vi "PAQmem_WriteAll.vi"(8 "error in (no error)":errorcluster, 10 "BinHistData":T1, 11 "PAQ-memory in":refnum<class "PAQ-memory.lvclass">) -> (0 "error out":errorcluster, 3 "PAQ-memory out":refnum<class "PAQ-memory.lvclass">)   [LabVIEW 2020, in "PAQ-memory.lvclass"]
doc: "PAQ memory action: write one whole layer content (of multiple TAGs)\n\nThis VI writes fetched data from the database to the computer memory DVR element"
uses:
  PAQ-memory.lvclass
  DBAL/controls/BIN/BINdata.ctl
  PAQ-memory.lvclass/PAQ-memory.ctl
  DBAL/DBAL-BIN.lvclass
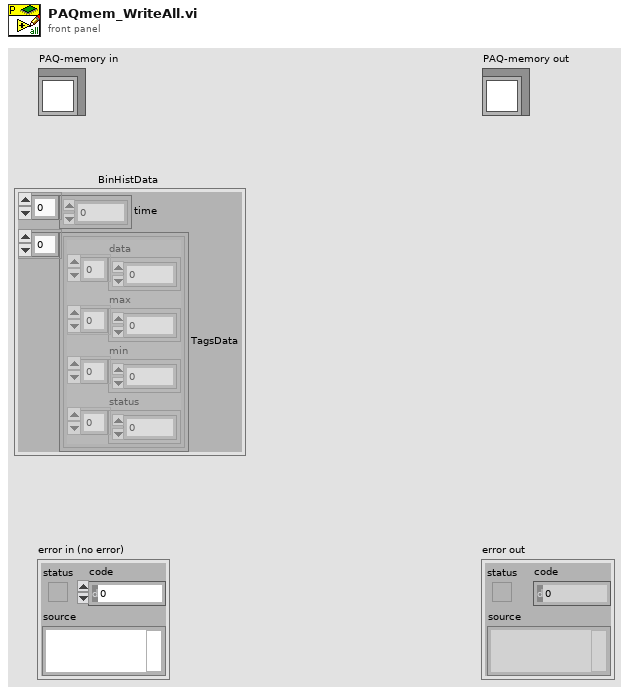
[diagram p1: front panel]
types:
  T1 = typedef "DBAL-BIN.lvclass/BINdata.ctl" = cluster{"time":dbl[], "TagsData":cluster{"data":dbl[], "max":dbl[], "min":dbl[], "status":u32[]}[]}
  T2 = cluster{"data":dbl[], "max":dbl[], "min":dbl[], "status":u32[]}[]
  T3 = cluster{"source":refnum<data-value>, "status":refnum<data-value>, "data":refnum<data-value>, "max":refnum<data-value>, "min":refnum<data-value>}[]
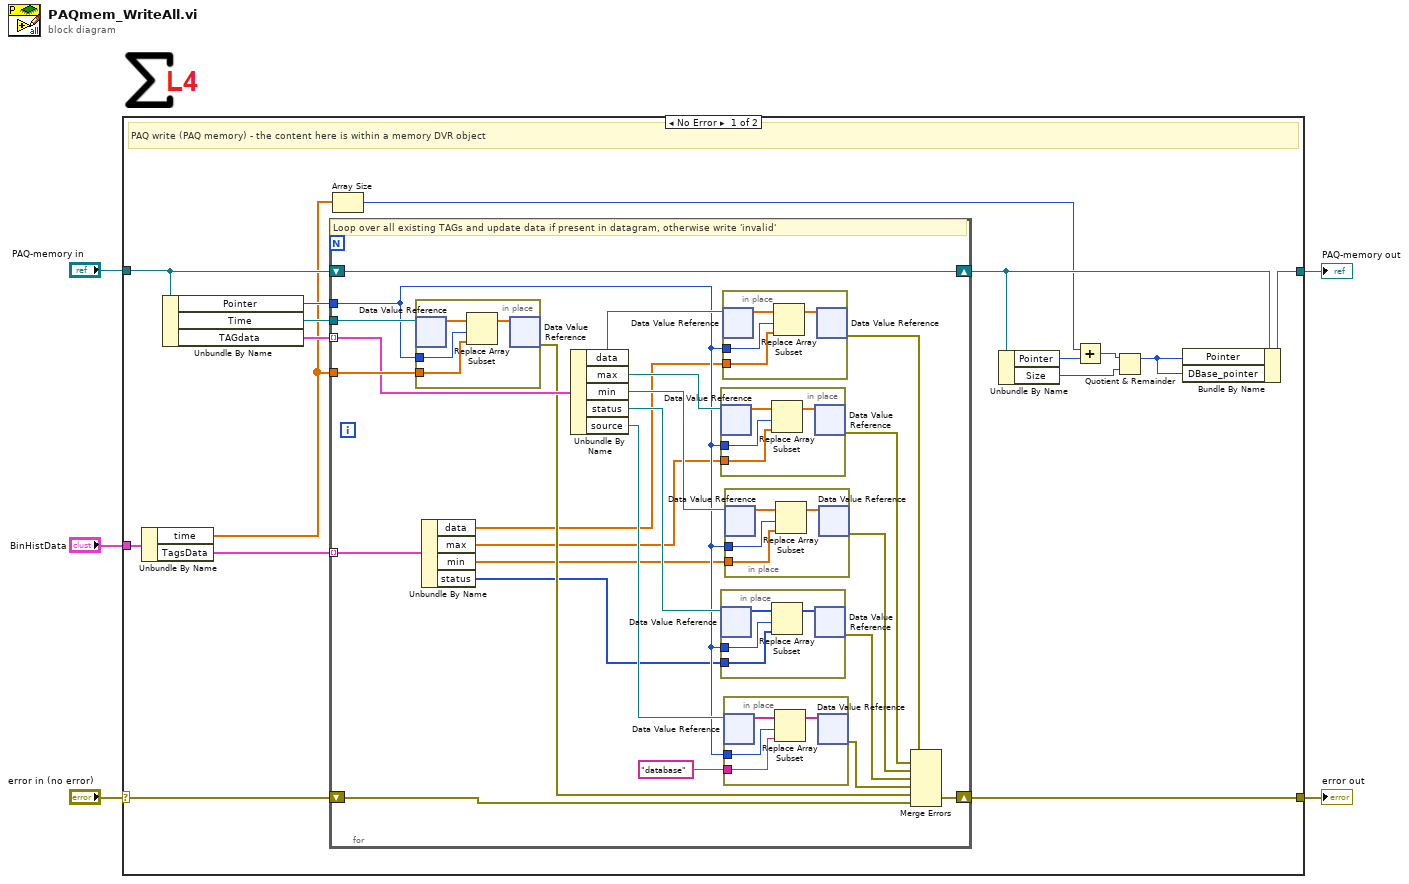
[diagram p0: block diagram]
diagram:
  n1 = case shown="No Error" "error in (no error)" {
    selector: "error in (no error)" -> [w21 w71]
    tunnel: [w20 w71] -> w4
    tunnel: [w13 w70] -> w2
    tunnel: "PAQ-memory in" -> [w19 w70]
    tunnel: "BinHistData" -> [w12 _]
    frame No Error {
      # "PAQ write (PAQ memory) - the content here is within a memory DVR object"
      n2 = Unbundle By Name(w12) -> ("time"=w10:dbl[], "TagsData"=w11:T2)
      n3 = Unbundle By Name(w19) -> ("Pointer"=w18:i32, "Time"=w17:refnum<data-value>, "TAGdata"=w16:T3)
      n4 = for {
        tunnel: w10 -> [w43]
        shift-right: [w33] -> w20
        shift-left: w21 -> [w35]
        shift-right: [w45] -> w14
        shift-left: w19 -> [w45]
        tunnel: w18 -> [w36]
        tunnel: w17 -> [w44]
        tunnel: w16 -> [w42] mode=indexing
        tunnel: w11 -> [w26] mode=indexing
        # "Loop over all existing TAGs and update data if present in datagram, otherwise write 'invalid'"
        n5 = in-place {
          in-place-border: w36 -> [w67]
          in-place-border: w43 -> [w66]
          n6 = in-place-dvr #1(w44) -> (w69:dbl[])  [unwired: 1 out]
          n7 = Replace Array Subset(array=w69, new element=w66, index=w67) -> (w68:dbl[])
          n8 = in-place-dvr #1(w68) -> (w28:errorcluster)  [unwired: 1 out]
        }
        n9 = Unbundle By Name(w26) -> ("data"=w25:dbl[], "max"=w24:dbl[], "min"=w23:dbl[], "status"=w22:u32[])
        n10 = Unbundle By Name(w42) -> ("data"=w41:refnum<data-value>, "max"=w40:refnum<data-value>, "min"=w39:refnum<data-value>, "status"=w38:refnum<data-value>, "source"=w37:refnum<data-value>)
        n11 = in-place {
          in-place-border: w36 -> [w59]
          in-place-border: w24 -> [w58]
          n12 = in-place-dvr #2(w40) -> (w61:dbl[])  [unwired: 1 out]
          n13 = Replace Array Subset(array=w61, new element=w58, index=w59) -> (w60:dbl[])
          n14 = in-place-dvr #2(w60) -> (w32:errorcluster)  [unwired: 1 out]
        }
        n15 = in-place {
          in-place-border: w36 -> [w51]
          in-place-border: w22 -> [w50]
          n16 = in-place-dvr #3(w38) -> (w53:u32[])  [unwired: 1 out]
          n17 = Replace Array Subset(array=w53, new element=w50, index=w51) -> (w52:u32[])
          n18 = in-place-dvr #3(w52) -> (w30:errorcluster)  [unwired: 1 out]
        }
        n19 = in-place {
          in-place-border: w36 -> [w63]
          in-place-border: w25 -> [w62]
          n20 = in-place-dvr #4(w41) -> (w65:dbl[])  [unwired: 1 out]
          n21 = Replace Array Subset(array=w65, new element=w62, index=w63) -> (w64:dbl[])
          n22 = in-place-dvr #4(w64) -> (w34:errorcluster)  [unwired: 1 out]
        }
        n23 = in-place {
          in-place-border: w36 -> [w47]
          in-place-border: "database" -> [w46]
          n24 = in-place-dvr #5(w37) -> (w49:string[])  [unwired: 1 out]
          n25 = Replace Array Subset(array=w49, new element=w46, index=w47) -> (w48:string[])
          n26 = in-place-dvr #5(w48) -> (w29:errorcluster)  [unwired: 1 out]
        }
        n27 = in-place {
          in-place-border: w36 -> [w55]
          in-place-border: w23 -> [w54]
          n28 = in-place-dvr #6(w39) -> (w57:dbl[])  [unwired: 1 out]
          n29 = Replace Array Subset(array=w57, new element=w54, index=w55) -> (w56:dbl[])
          n30 = in-place-dvr #6(w56) -> (w31:errorcluster)  [unwired: 1 out]
        }
        n31 = Merge Errors(w34, w32, w31, w30, w29, w28, w35) -> (w33:errorcluster)
      }
      n32 = Array Size(array=w10) -> (size(s)=w8:i32)
      n33 = Unbundle By Name(w14) -> ("Pointer"=w9:i32, "Size"=w15:i32)
      n34 = Add(x=w8, y=w9) -> (x+y=w7:i32)
      n35 = Quotient & Remainder(x=w7, y=w15) -> (x-y*floor(x/y)=w6:i32)  [unwired: 1 out]
      n36 = Bundle By Name(cluster=w14, "Pointer"=w6, "DBase_pointer"=w6) -> (w13:refnum<class "PAQ-memory.lvclass">)
    }
    frame Error {
    }
  }
  "error out" <- w4
  "PAQ-memory out" <- w2
